vi "Read dblEventParams.vi"(8 "error in (no error)":errorcluster, 11 "PmuImpairPluginBase in":refnum<class "PmuImpairPluginBase.lvclass">) -> (0 "error out":errorcluster, 2 "dblEventParams":dbl[][](array[numeric]), 3 "PmuImpairPluginBase out":refnum<class "PmuImpairPluginBase.lvclass">)   [LabVIEW 2014, in "PmuImpairPlugins.lvlib" / "PmuImpairPluginBase.lvclass"]
uses:
  PmuImpairPluginBase.lvclass
  PmuImpairPluginBase.lvclass/PmuImpairPluginBase.ctl
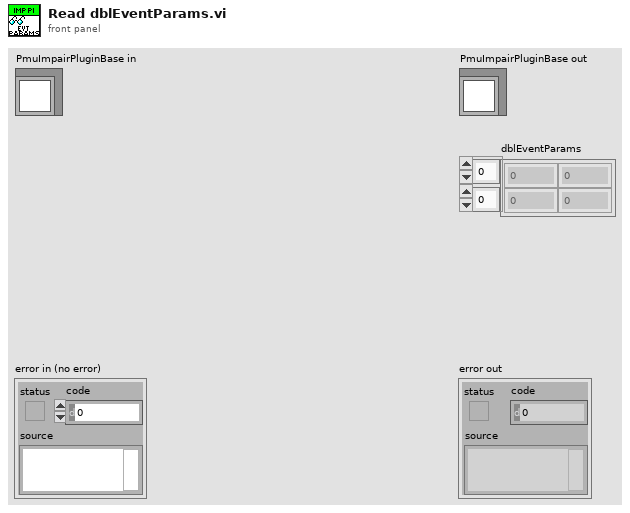
[diagram p1: front panel]
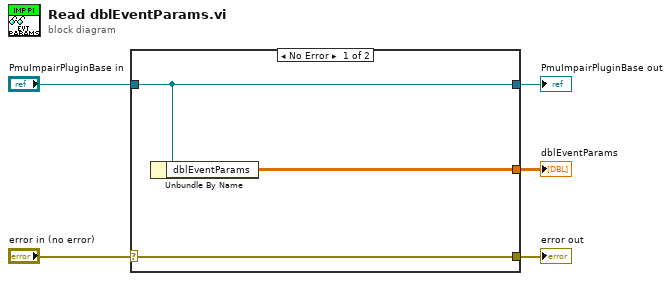
[diagram p0: block diagram]
diagram:
  n1 = case shown="No Error" "error in (no error)" {
    selector: "error in (no error)" -> [w8 w9]
    tunnel: [w8 w9] -> w4
    tunnel: [w7 w10] -> w2
    tunnel: "PmuImpairPluginBase in" -> [w7 w10]
    tunnel: [w6 _] -> w1
    frame No Error {
      n2 = Unbundle By Name(w7) -> ("dblEventParams"=w6:dbl[][])
    }
    frame Error {
    }
  }
  "error out" <- w4
  "PmuImpairPluginBase out" <- w2
  "dblEventParams" <- w1
